vi "_Yt08_Msgbox.vi"(11 "YTESTER测试数据":T1 caption="不要修改！") -> (3 "YTESTER结论":T2)   [LabVIEW 2017]
doc: "VIDescription=弹出一个简单的信息框，支持三个按钮及图片！\nVIClassID=YT_SSTEPFLAG_MSGBOX"
uses:
  YtCommon.lvlibp/yt`Step StepBaseInput.ctl
  Step`s VIs/YYLLIdea/yylltestresult/yylltestresult basis.ctl
  YtCommon.lvlibp/yt`Step StepResult.ctl
  YtCommon.lvlibp/yt`Step TestData.ctl
  YtCommon.lvlibp/yt`Step System Queue.ctl
  Step`s VIs/YYLLGeneric/variable_W.ctl
  YtCommon.lvlibp/yt`Data-Ytester Type Data.ctl
  YtCommon.lvlibp
panel:
  in  "YTESTER开放参数":T5={"YTESTER_BaseInput"={"isTest"=FALSE, "isSkip"=FALSE, "StepName"="消息", "OnPass"=enum."Next", "OnFail"=enum."Next", "ReTestNumber"=0.0}, "消息标题"="", "消息内容"="", "消息存在时间（s）"=0.0, "不允许关闭消息框（消息时间大于0）"=FALSE, "左边按钮文本"="", "中间按钮文本"="OK", "右边按钮文本"="", "聚焦按钮"=enum."Btn2", "合格依据"=enum."强制合格", "StringLimit-A"="", "UpperLimit-B"=0.0, "LowLimit-C"=0.0, "unit"="", "JPG-PNG-BMP 图片Path"=path "", "按下按钮的文本到变量(自定义建议#开头)"="不到变量"}
  # "消息框"
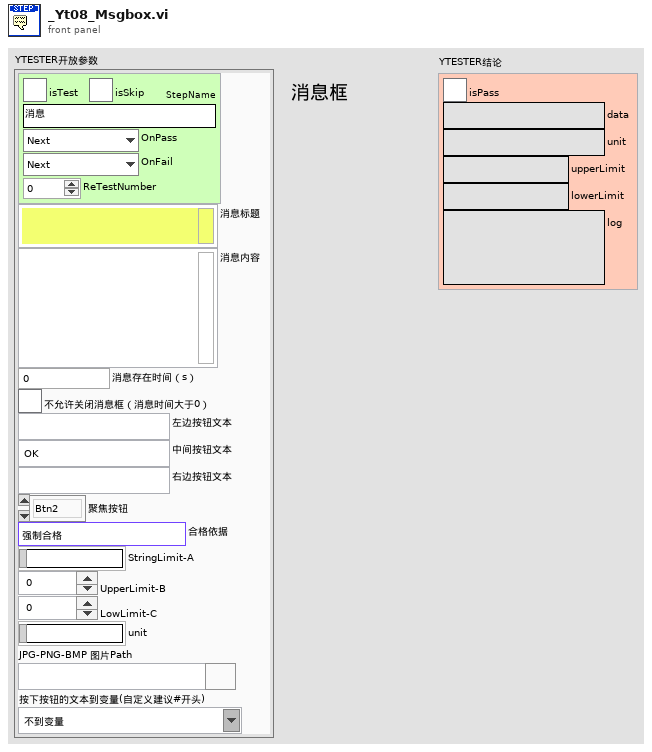
[diagram p1: front panel]
types:
  T1 = typedef "YtCommon.lvlibp/yt`Step TestData.ctl" = cluster{"Socket(From1)":i32, "SN":refnum<notifier>, "StopFlagRef":refnum<notifier>, "YT System Queue":refnum<queue>}
  T2 = typedef "YtCommon.lvlibp/yt`Step StepResult.ctl" = cluster{"isPass":bool, "data":string, "unit":string, "upperLimit":string, "lowerLimit":string, "log":string}
  T3 = typedef "YtCommon.lvlibp/yt`Step StepBaseInput.ctl" = cluster{"isTest":bool, "isSkip":bool, "StepName":string, "OnPass":enum16{"Next", "ToOVER", "Terminate"}, "OnFail":enum16{"Next", "ToOVER", "Terminate"}, "ReTestNumber":dbl}
  T4 = typedef "yylltestresult basis.ctl" = enum16{"强制合格", "强制不合格", "随机合格", "X=A", "X=\"真\"", "X=\"假\"", "X≠A", "X包含A", "X不包含A", "A包含X", "A包含非空X", "A不包含X", "X等于A正则匹配内容", "X包含A正则匹配内容", "X不包含A正则匹配内容", "X=B", "X≠B", "X＞B", "X≥B", "X＜B", "X≤B", "B≥X≥C", "B≥X＞C", "B＞X≥C", "B＞X＞C", "X≥B | C≥X", "X＞B | C≥X", "X≥B | C＞X", "X＞B | C＞X"}
  T5 = cluster{"YTESTER_BaseInput":T3, "消息标题":string, "消息内容":string, "消息存在时间（s）":dbl, "不允许关闭消息框（消息时间大于0）":bool, "左边按钮文本":string, "中间按钮文本":string, "右边按钮文本":string, "聚焦按钮":enum16{"无", "Btn1", "Btn2", "Btn3"}, "合格依据":T4, "StringLimit-A":string, "UpperLimit-B":dbl, "LowLimit-C":dbl, "unit":string, "JPG-PNG-BMP 图片Path":path, "按下按钮的文本到变量(自定义建议#开头)":string}
  T6 = typedef "variable_W.ctl" = cluster{"YT_TYPE":T7, "TypeData":string[], "Tips":string}
  T7 = typedef "YtCommon.lvlibp/yt`Data-Ytester Type Data.ctl" = enum16{"NULL", "NUM", "BOOL", "TXT", "ENUM", "TIME", "PATH", "VISA", "COMBO", "ColorBox", "RadioBtn", "Array_NUM", "Array_BOOL", "Array_TXT", "Array_ENUM", "Array_PATH", "Array_COMBO"}
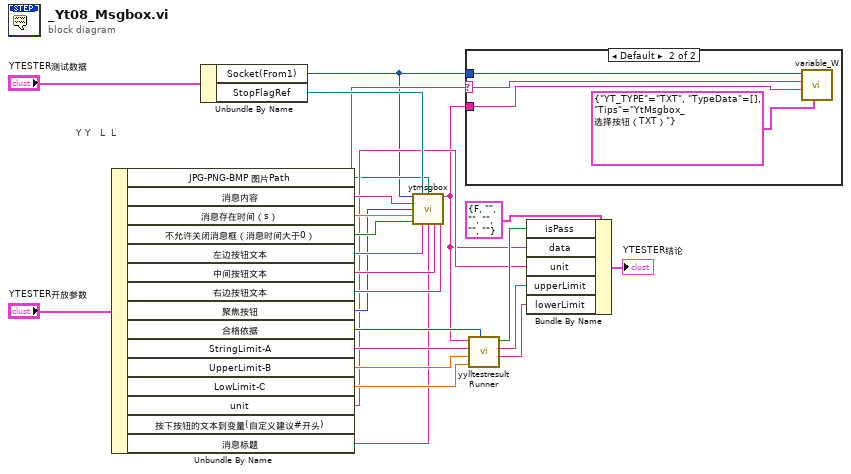
[diagram p0: block diagram]
diagram:
  # "Y Y   L  L"
  n1 = Unbundle By Name("YTESTER开放参数") -> ("JPG-PNG-BMP 图片Path"=w5:path, "消息内容"=w21:string, "消息存在时间（s）"=w20:dbl, "不允许关闭消息框（消息时间大于0）"=w19:bool, "左边按钮文本"=w17:string, "中间按钮文本"=w16:string, "右边按钮文本"=w15:string, "聚焦按钮"=w14:enum16{"无", "Btn1", "Btn2", "Btn3"}, "合格依据"=w12:T4, "StringLimit-A"=w11:string, "UpperLimit-B"=w10:dbl, "LowLimit-C"=w9:dbl, "unit"=w6:string, "按下按钮的文本到变量(自定义建议#开头)"=w4:string, "消息标题"=w1:string)
  n2 = Unbundle By Name("YTESTER测试数据") -> ("Socket(From1)"=w3:i32, "StopFlagRef"=w18:refnum<notifier>)
  n3 = call "ytmsgbox.vi"("Socket(From1)"=w3, "StopFlagRef"=w18, "JPEGPNGBMP file"=w5, "String"=w21, "聚焦"=w14, "消息存在时间（s）"=w20, "不可关闭"=w19, "按钮1文本"=w17, "Title"=w1, "按钮2文本"=w16, "按钮3文本"=w15) -> ("BtnSelectOut"=w2:string)  [unwired: 4 in]
  n4 = case shown="Default" w4 {
    selector: w4 -> [_ w28]
    tunnel: w3 -> [_ w29]
    tunnel: w2 -> [_ w27]
    frame "不到变量" {
    }
    frame Default {
      n5 = call "variable_W.vi"("附加的Information"=T6 {"YT_TYPE"=enum."TXT", "TypeData"=[], "Tips"="YtMsgbox_选择按钮（TXT）"}, "待写入池的输入控件"=w27, "待写入池变量名称"=w28, "函数池名称 in"=w29) -> ()  [unwired: 5 in, 3 out]
    }
  }
  n6 = call "yylltestresult Runner.vi"("合格依据"=w12, "LowLimit-C"=w9, "UpperLimit-B"=w10, "StringLimit-A"=w11, "DataIn-X"=w2) -> ("lowerLimit"=w8:string, "upperLimit"=w7:string, "isPass"=w13:bool)  [unwired: 4 in]
  n7 = Bundle By Name(cluster=T2 {"isPass"=FALSE, "data"="", "unit"="", "upperLimit"="", "lowerLimit"="", "log"=""} ("Result"), "isPass"=w13, "data"=w2, "unit"=w6, "upperLimit"=w7, "lowerLimit"=w8) -> (→"YTESTER结论":T2)
